vi "LabVIEW Calculator.vi"() -> ()   [LabVIEW 2022 SP3]
panel:
  out "Calculator Display":string
  in  "Calculator UI":T1
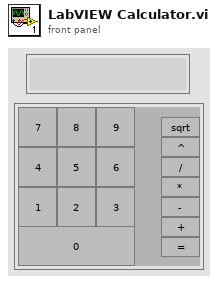
[diagram p1: front panel]
types:
  T1 = cluster{"0":bool, "6":bool, "7":bool, "8":bool, "9":bool, "3":bool, "4":bool, "5":bool, "1":bool, "2":bool, "Multiply":bool, "Divide":bool, "Subtract":bool, "Add":bool, "Result":bool, "sqrt":bool, "Power":bool}
  T2 = enum16{"No Function", "Add", "Subtract", "Multiply", "Divide", "sqrt", "Power"}
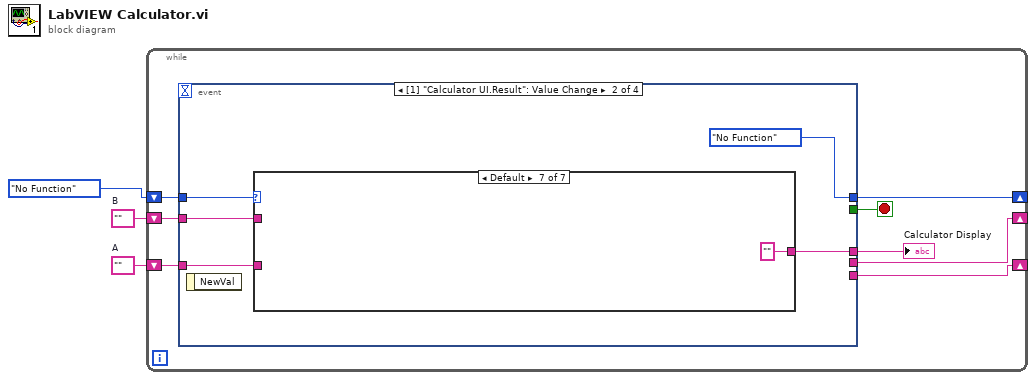
[diagram p0: block diagram]
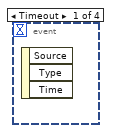
[diagram p2: hidden frame]
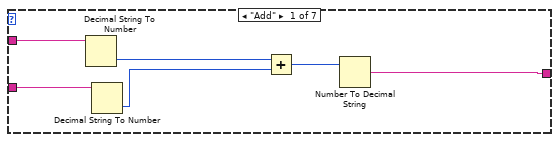
[diagram p3: hidden frame]
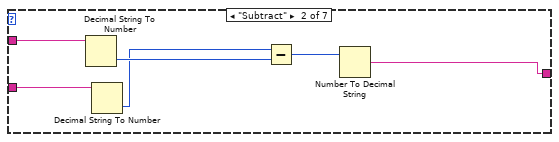
[diagram p4: hidden frame]
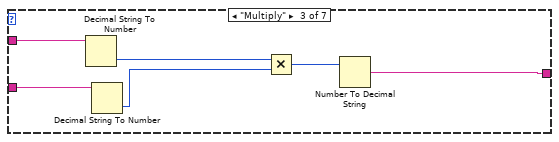
[diagram p5: hidden frame]
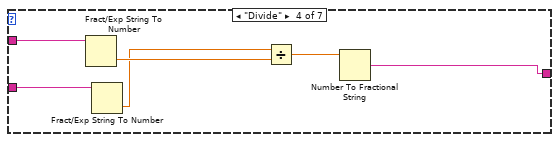
[diagram p6: hidden frame]
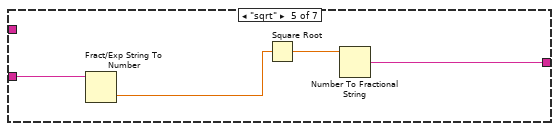
[diagram p7: hidden frame]
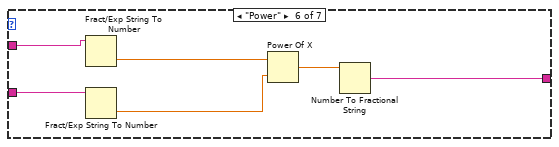
[diagram p8: hidden frame]
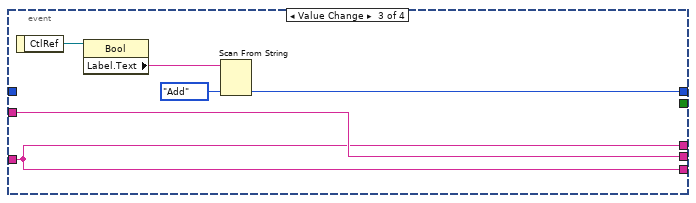
[diagram p9: hidden frame]
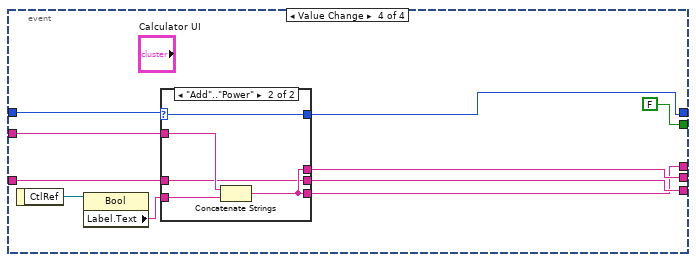
[diagram p10: hidden frame]
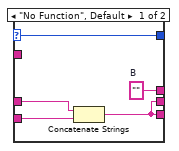
[diagram p11: hidden frame]
diagram:
  w2 = ""  # A
  w3 = ""  # B
  n1 = while {
    shift-right: [w7] -> _
    shift-left: w3 -> [w11]
    shift-right: [w8] -> _
    shift-left: w2 -> [w10]
    shift-right: [w4] -> _
    shift-left: T2."No Function" -> [w9]
    stop <- w5 stop-if-true
    n2 = event shown="[1] \"Calculator UI.Result\": Value Change" {
      selector: _ -> [_ _ _ _]
      dyn-events: _ -> [_ _ _ _]
      timeout: _ -> [_ _ _ _]
      tunnel: w11 -> [_ w15 w55 w65]
      tunnel: w10 -> [_ w14 w53 w63]
      tunnel: w9 -> [_ w13 _ w61]
      tunnel: [_ _ w53 w59] -> w8
      tunnel: [_ _ w55 w62] -> w7
      tunnel: [_ w16 w53 w58] -> w6
      tunnel: [_ _ _ FALSE] -> w5
      tunnel: [_ T2."No Function" w54 w60] -> w4
      event Timeout {
        n3 = event-data() -> ()  [unwired: 1 in, 3 out]
      }
      event "Calculator UI.Result": Value Change {
        n4 = event-data() -> ()  [unwired: 1 in, 1 out]
        n5 = case shown="Default" w13 {
          tunnel: w15 -> [w22 w28 w34 w40 _ w50 _]
          tunnel: w14 -> [w21 w27 w33 w39 w41 w49 _]
          tunnel: [w17 w23 w29 w35 w42 w46 ""] -> w16
          frame "Add" {
            n6 = Decimal String To Number(string=w22) -> (number=w20:i32)  [unwired: 2 in, 1 out]
            n7 = Decimal String To Number(string=w21) -> (number=w19:i32)  [unwired: 2 in, 1 out]
            n8 = Add(x=w20, y=w19) -> (x+y=w18:i32)
            n9 = Number To Decimal String(number=w18) -> (decimal integer string=w17:string)  [unwired: 1 in]
          }
          frame "Subtract" {
            n10 = Decimal String To Number(string=w28) -> (number=w26:i32)  [unwired: 2 in, 1 out]
            n11 = Decimal String To Number(string=w27) -> (number=w25:i32)  [unwired: 2 in, 1 out]
            n12 = Subtract(x=w25, y=w26) -> (x-y=w24:i32)
            n13 = Number To Decimal String(number=w24) -> (decimal integer string=w23:string)  [unwired: 1 in]
          }
          frame "Multiply" {
            n14 = Decimal String To Number(string=w34) -> (number=w32:i32)  [unwired: 2 in, 1 out]
            n15 = Decimal String To Number(string=w33) -> (number=w31:i32)  [unwired: 2 in, 1 out]
            n16 = Multiply(x=w32, y=w31) -> (x*y=w30:i32)
            n17 = Number To Decimal String(number=w30) -> (decimal integer string=w29:string)  [unwired: 1 in]
          }
          frame "Divide" {
            n18 = Fract/Exp String To Number(string=w40) -> (number=w38:dbl)  [unwired: 3 in, 1 out]
            n19 = Fract/Exp String To Number(string=w39) -> (number=w37:dbl)  [unwired: 3 in, 1 out]
            n20 = Divide(x=w37, y=w38) -> (x/y=w36:dbl)
            n21 = Number To Fractional String(number=w36) -> (F-format string=w35:string)  [unwired: 3 in]
          }
          frame "sqrt" {
            n22 = Fract/Exp String To Number(string=w41) -> (number=w44:dbl)  [unwired: 3 in, 1 out]
            n23 = Square Root(x=w44) -> (sqrt(x)=w43:dbl)
            n24 = Number To Fractional String(number=w43) -> (F-format string=w42:string)  [unwired: 3 in]
          }
          frame "Power" {
            n25 = Fract/Exp String To Number(string=w50) -> (number=w48:dbl)  [unwired: 3 in, 1 out]
            n26 = Fract/Exp String To Number(string=w49) -> (number=w47:dbl)  [unwired: 3 in, 1 out]
            n27 = Power Of X(1:w47, 2:w48) -> (0:w45:dbl)
            n28 = Number To Fractional String(number=w45) -> (F-format string=w46:string)  [unwired: 3 in]
          }
          frame Default {
          }
        }
      }
      event "Calculator UI.Multiply", "Calculator UI.Divide", "Calculator UI.Subtract", "Calculator UI.Add", "Calculator UI.sqrt", "Calculator UI.Power": Value Change {
        n29 = event-data() -> ("CtlRef"=w56:refnum<vi>)  [unwired: 1 in]
        n30 = property class="Bool"(reference=w56) -> ("Label.Text"=w57:string)  [unwired: 1 in, 2 out]
        n31 = Scan From String "Scan From String"(input string=w57, default 1=T2."Add") -> (output 1=w54:T2)  [unwired: 3 in, 3 out]
      }
      event "Calculator UI.0", "Calculator UI.1", "Calculator UI.2", "Calculator UI.3", "Calculator UI.4", "Calculator UI.5", "Calculator UI.6", "Calculator UI.7", "Calculator UI.8", "Calculator UI.9": Value Change {
        n32 = event-data() -> ("CtlRef"=w67:refnum<vi>)  [unwired: 1 in]
        n33 = property class="Bool"(reference=w67) -> ("Label.Text"=w64:string)  [unwired: 1 in, 2 out]
        n34 = case shown="\"Add\"..\"Power\"" w61 {
          selector: w61 -> [w72 w77]
          tunnel: [w72 w77] -> w60
          tunnel: [w71 w74] -> w62
          tunnel: [w70 w74] -> w58
          tunnel: [w70 w73] -> w59
          tunnel: w65 -> [_ w76]
          tunnel: w64 -> [w68 w75]
          tunnel: w63 -> [w69 w73]
          frame "No Function", Default {
            w71 = ""  # B
            n35 = Concatenate Strings(w69, w68) -> (w70:string)
          }
          frame "Add".."Power" {
            n36 = Concatenate Strings(w76, w75) -> (w74:string)
          }
        }
      }
    }
    "Calculator Display" <- w6
  }
